vi "serial port init.vi"(8 "错误输入（无错误）":errorcluster, 10 "海马(1)":bool, 11 "VISA引用句柄输入":refnum<visa-resource-name>="COM1") -> (0 "错误输出":errorcluster, 3 "VISA引用句柄输出":refnum<visa-resource-name>)   [LabVIEW 2013]
uses:
  C:/Program Files/National Instruments/LabVIEW 2013/examples/Instrument IO/Serial/support/Serial - Settings.ctl
  <vilib>/Instr/_visa.llb/VISA Flush IO Buffer Mask.ctl
  <vilib>/Instr/_visa.llb/VISA Configure Serial Port (Instr).vi
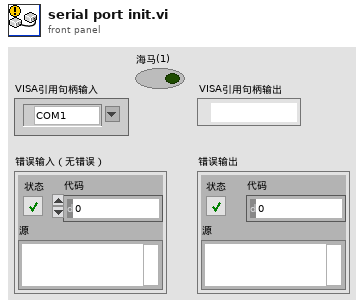
[diagram p1: front panel]
types:
  T1 = typedef "Serial - Settings.ctl" = cluster{"波特率":u32, "数据比特":u16, "奇偶":enum16{"None", "Odd", "Even", "Mark", "Space"}, "停止位":u16, "流控制":u16}
  T2 = typedef "VISA Flush IO Buffer Mask.ctl" = u16
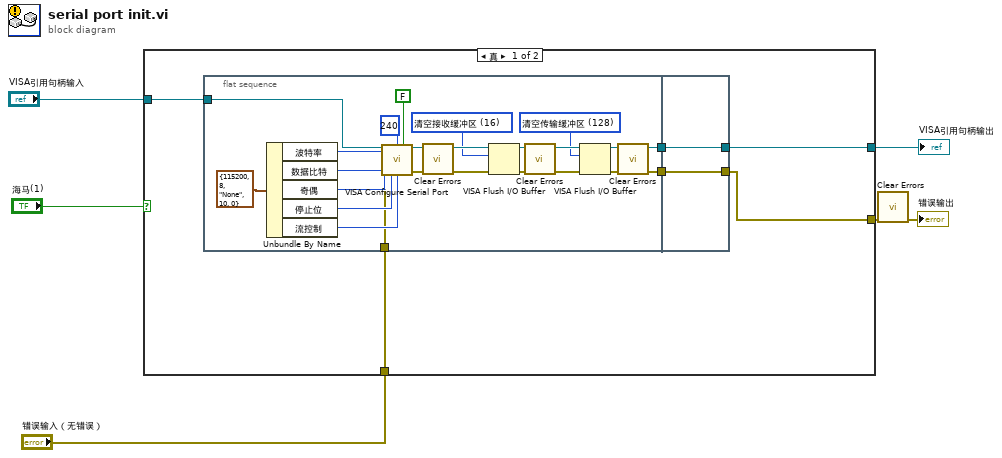
[diagram p0: block diagram]
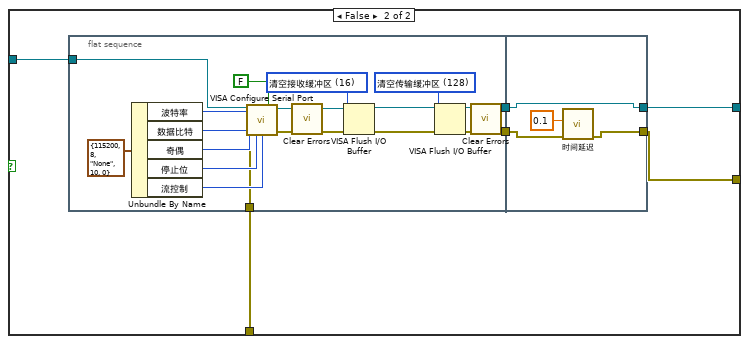
[diagram p2: hidden frame]
diagram:
  n1 = case shown="真" "海马(1)" {
    tunnel: [w10 w40] -> w6
    tunnel: [w9 w39] -> w5
    tunnel: "错误输入（无错误）" -> [w8 w38]
    tunnel: "VISA引用句柄输入" -> [w7 w37]
    frame True {
      n2 = flat-sequence {
        tunnel: w8 -> [w27]
        tunnel: [w21] -> w12
        tunnel: [w13] -> w11
        tunnel: w7 -> [w24]
        tunnel: [w34] -> w10
        tunnel: [w35] -> w9
        tunnel: w12 -> [w35]
        tunnel: w11 -> [w34]
        frame #0 {
          w16 = T2 128 items=["清空接收缓冲区"=16, "向设备写入传输缓冲区"=32, "清空接收缓冲区（无I/O）"=64, "清空传输缓冲区"=128] ("Mask")
          w17 = T2 16 items=["清空接收缓冲区"=16, "向设备写入传输缓冲区"=32, "清空接收缓冲区（无I/O）"=64, "清空传输缓冲区"=128] ("Mask")
          n3 = Unbundle By Name(T1 {"波特率"=115200, "数据比特"=8, "奇偶"=enum."None", "停止位"=10, "流控制"=0} ("串口设置")) -> ("波特率"=w30:u32, "数据比特"=w31:u16, "奇偶"=w32:enum16{"None", "Odd", "Even", "Mark", "Space"}, "停止位"=w33:u16, "流控制"=w28:u16)
          n4 = call-poly "VISA Configure Serial Port"("VISA resource name"=w24, "termination char\n(0xA = '\\n' = LF)"=u8 240 ("termination char\n(0xA = '\\n' = LF)"), "Enable Termination\nChar (T)"=FALSE ("Enable Termination\nChar (T)"), "baud rate (9600)"=w30, "data bits (8)"=w31, "parity (0:none)"=w32, "error in (no error)"=w27, "stop bits (10: 1 bit)"=w33, "flow control (0:none)"=w28) -> ("VISA resource name out"=w18:refnum<visa-resource-name>, "error out"=w19:errorcluster)  [unwired: 1 in, 4 out]
          n5 = call <vilib>:"Clear Errors.vi"("error in (no error)"=w19) -> ("error out"=w15:errorcluster)  [unwired: 6 in]
          n6 = VISA Flush I/O Buffer(VISA resource name=w18, mask (16)=w17, error in (no error)=w15) -> (VISA resource name out=w22:refnum<visa-resource-name>, error out=w23:errorcluster)
          n7 = call <vilib>:"Clear Errors.vi"("error in (no error)"=w23) -> ("error out"=w14:errorcluster)  [unwired: 6 in]
          n8 = VISA Flush I/O Buffer(VISA resource name=w22, mask (16)=w16, error in (no error)=w14) -> (VISA resource name out=w21:refnum<visa-resource-name>, error out=w20:errorcluster)
          n9 = call <vilib>:"Clear Errors.vi"("error in (no error)"=w20) -> ("error out"=w13:errorcluster)  [unwired: 6 in]
        }
        frame #1 {
        }
      }
    }
    frame False {
      n10 = flat-sequence {
        tunnel: w38 -> [w54]
        tunnel: [w47] -> w41
        tunnel: w37 -> [w51]
        tunnel: [w42] -> w36
        tunnel: [w61] -> w40
        tunnel: [w62] -> w39
        tunnel: w41 -> [w62]
        tunnel: w36 -> [w63]
        frame #0 {
          w45 = T2 128 items=["清空接收缓冲区"=16, "向设备写入传输缓冲区"=32, "清空接收缓冲区（无I/O）"=64, "清空传输缓冲区"=128] ("Mask")
          w50 = T2 16 items=["清空接收缓冲区"=16, "向设备写入传输缓冲区"=32, "清空接收缓冲区（无I/O）"=64, "清空传输缓冲区"=128] ("Mask")
          n11 = Unbundle By Name(T1 {"波特率"=115200, "数据比特"=8, "奇偶"=enum."None", "停止位"=10, "流控制"=0} ("串口设置")) -> ("波特率"=w57:u32, "数据比特"=w58:u16, "奇偶"=w59:enum16{"None", "Odd", "Even", "Mark", "Space"}, "停止位"=w60:u16, "流控制"=w55:u16)
          n12 = call-poly "VISA Configure Serial Port"("VISA resource name"=w51, "Enable Termination\nChar (T)"=FALSE ("Enable Termination\nChar (T)"), "baud rate (9600)"=w57, "data bits (8)"=w58, "parity (0:none)"=w59, "error in (no error)"=w54, "stop bits (10: 1 bit)"=w60, "flow control (0:none)"=w55) -> ("VISA resource name out"=w52:refnum<visa-resource-name>, "error out"=w53:errorcluster)  [unwired: 2 in, 4 out]
          n13 = call <vilib>:"Clear Errors.vi"("error in (no error)"=w53) -> ("error out"=w43:errorcluster)  [unwired: 6 in]
          n14 = VISA Flush I/O Buffer(VISA resource name=w52, mask (16)=w50, error in (no error)=w43) -> (VISA resource name out=w48:refnum<visa-resource-name>, error out=w49:errorcluster)
          n15 = VISA Flush I/O Buffer(VISA resource name=w48, mask (16)=w45, error in (no error)=w49) -> (VISA resource name out=w47:refnum<visa-resource-name>, error out=w46:errorcluster)
          n16 = call <vilib>:"Clear Errors.vi"("error in (no error)"=w46) -> ("error out"=w42:errorcluster)  [unwired: 6 in]
        }
        frame #1 {
          n17 = call "时间延迟"("error in (no error)"=w63, "Delay Time (s)"=0.1) -> ("error out"=w61:errorcluster)  [unwired: 9 in]
        }
      }
    }
  }
  "VISA引用句柄输出" <- w5
  n18 = call <vilib>:"Clear Errors.vi"("error in (no error)"=w6) -> ("error out"=→"错误输出":errorcluster)  [unwired: 6 in]
